vi "Write to File.vi"(7 "Section Name":string, 8 "error in (no error)":errorcluster, 10 "INI Ref":T1, 11 "Boolean Assertion in":refnum<class "Boolean Assertion.lvclass">) -> (0 "error out":errorcluster, 2 "INI Ref out":T1, 3 "Boolean Assertion out":refnum<class "Boolean Assertion.lvclass">)   [LabVIEW 2020, in "MacroAssert.lvlib" / "Boolean Assertion.lvclass"]
doc: "Writes associated parameters to the file identified by <B>INI Ref</B>."
uses:
  Boolean Assertion.lvclass
  <vilib>/Utility/config.llb/Config Data RefNum.ctl
  <vilib>/Utility/error.llb/Error Cluster From Error Code.vi
  <vilib>/Utility/config.llb/Write Key (String).vi
  <vilib>/Utility/config.llb/Write Key (Boolean).vi
  Assertion Step/Assertion Step.lvclass
  MacroAssert.lvlib
  <vilib>/Utility/config.llb/NI_LVConfig.lvlib
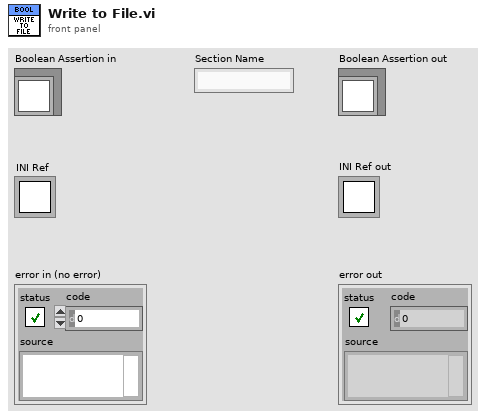
[diagram p1: front panel]
types:
  T1 = typedef "NI_LVConfig.lvlib/Config Data RefNum.ctl" = refnum<k1>
  T2 = typedef "MacroAssert.lvlib/Boolean Assertion.lvclass/Boolean Assertion Type.ctl" = enum16{"Boolean Ctl Value", "Ctl Visible Property", "Ctl is Enabled", "Ctl is Grayed Out", "Ctl Key Focus Property", "Window is in Running Windows", "VI Front Panel is Open"}
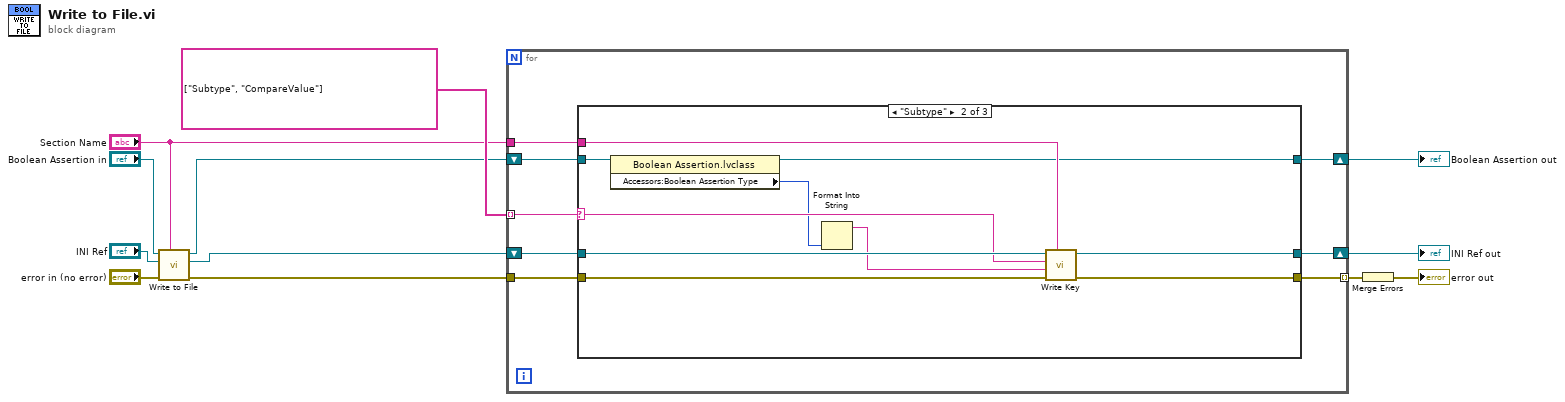
[diagram p0: block diagram]
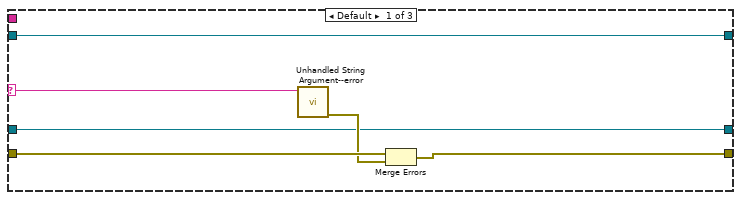
[diagram p2: hidden frame]
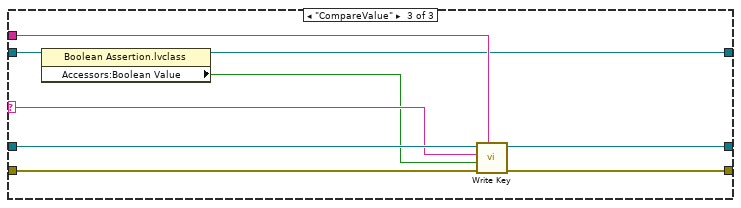
[diagram p3: hidden frame]
diagram:
  n1 = call-parent "Write to File.vi"("Section Name"="Section Name", "error in (no error)"="error in (no error)", "INI Ref"="INI Ref", "Assertion Step in"="Boolean Assertion in") -> ("error out"=w10:errorcluster, "INI Ref out"=w7:T1, "Assertion Step out"=w3:refnum<class "Boolean Assertion.lvclass">)  [unwired: 5 in]
  n2 = for {
    tunnel: string[] ["Subtype", "CompareValue"] -> [w16] mode=indexing
    tunnel: w10 -> [w20]
    tunnel: "Section Name" -> [w15]
    shift-right: [w13] -> w2
    shift-left: w3 -> [w14]
    tunnel: [w19] -> w4 mode=indexing
    shift-right: [w17] -> w8
    shift-left: w7 -> [w18]
    n3 = case shown="\"Subtype\"" w16 {
      selector: w16 -> [w21 w31 w40]
      tunnel: w20 -> [w26 w36 w45]
      tunnel: w15 -> [_ w32 w41]
      tunnel: w14 -> [w22 w30 w39]
      tunnel: [w22 w27 w38] -> w13
      tunnel: [w24 w35 w44] -> w19
      tunnel: w18 -> [w23 w34 w43]
      tunnel: [w23 w33 w42] -> w17
      frame Default {
        n4 = call "Unhandled String Argument--error.vi"("Argument"=w21) -> ("error out"=w25:errorcluster)  [unwired: 10 in]
        n5 = Merge Errors(w26, w25) -> (w24:errorcluster)
      }
      frame "Subtype" {
        n6 = property class="Boolean Assertion.lvclass"(reference=w30) -> (reference out=w27:refnum<class "Boolean Assertion.lvclass">, "Accessors:Boolean Assertion Type"=w29:T2)  [unwired: 1 in, 1 out]
        n7 = Format Into String(w29) -> (resulting string=w28:string)  [unwired: 3 in, 1 out]
        n8 = call-poly <vilib>:"Write Key.vi"("section"=w32, "error in (no error)"=w36, "value"=w28, "key"=w31, "refnum"=w34) -> ("error out"=w35:errorcluster, "refnum out"=w33:T1)  [unwired: 4 in, 1 out]
      }
      frame "CompareValue" {
        n9 = property class="Boolean Assertion.lvclass"(reference=w39) -> (reference out=w38:refnum<class "Boolean Assertion.lvclass">, "Accessors:Boolean Value"=w37:bool)  [unwired: 1 in, 1 out]
        n10 = call-poly <vilib>:"Write Key.vi"("section"=w41, "error in (no error)"=w45, "value"=w37, "key"=w40, "refnum"=w43) -> ("error out"=w44:errorcluster, "refnum out"=w42:T1)  [unwired: 4 in, 1 out]
      }
    }
  }
  "Boolean Assertion out" <- w2
  "INI Ref out" <- w8
  n11 = Merge Errors(w4) -> (→"error out":errorcluster)
